vi "SetMFCSetPoint.vi"(8 "Setpoint":dbl, 11 "MFC ID Number":i32) -> ()   [LabVIEW 2011]
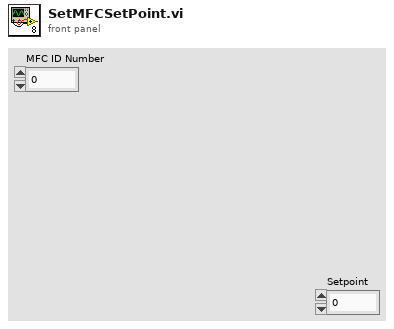
[diagram p1: front panel]
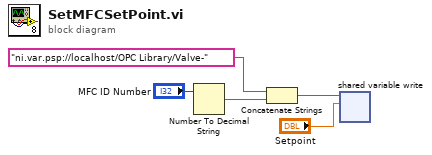
[diagram p0: block diagram]
diagram:
  n1 = Number To Decimal String(number="MFC ID Number") -> (decimal integer string=w5:string)  [unwired: 1 in]
  n2 = Concatenate Strings("ni.var.psp://localhost/OPC Library/Valve-", w5) -> (w3:string)
  n3 = shared-variable-write(w3, "Setpoint") -> ()  [unwired: 1 in, 2 out]
